vi "fpga_Reporting Rate Error Check (M Class).vi"(10 "reporting rate":i16, 11 "nominal frequency":enum16{"50 Hz", "60 Hz"}(ring)) -> (3 "error":i32)   [LabVIEW 2013, in "NI_EP_PMU_FPGA.lvlib"]
uses:
  <vilib>/addons/Electrical Power/PMU/NI_EP_PMU_FPGA.lvlib
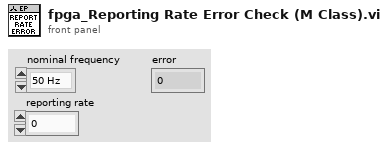
[diagram p1: front panel]
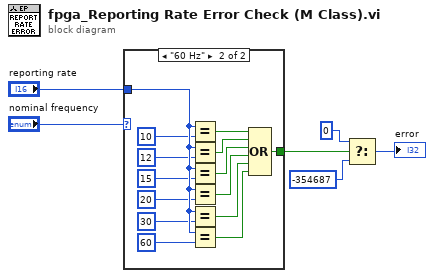
[diagram p0: block diagram]
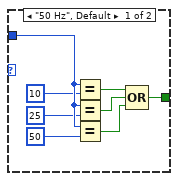
[diagram p2: hidden frame]
diagram:
  n1 = case shown="\"60 Hz\"" "nominal frequency" {
    tunnel: "reporting rate" -> [w11 w24]
    tunnel: [w10 w25] -> w4
    frame "50 Hz", Default {
      n2 = Equal?(x=w11, y=i16 10 ("reporting rate")) -> (x = y?=w14:bool)
      n3 = Equal?(x=w11, y=i16 25 ("reporting rate")) -> (x = y?=w13:bool)
      n4 = Equal?(x=w11, y=i16 50 ("reporting rate")) -> (x = y?=w12:bool)
      n5 = Compound Arithmetic op=OR(w14, w13, w12) -> (w10:bool)
    }
    frame "60 Hz" {
      n6 = Equal?(x=w24, y=i16 10 ("reporting rate")) -> (x = y?=w28:bool)
      n7 = Equal?(x=w24, y=i16 12 ("reporting rate")) -> (x = y?=w27:bool)
      n8 = Equal?(x=w24, y=i16 15 ("reporting rate")) -> (x = y?=w26:bool)
      n9 = Equal?(x=w24, y=i16 20 ("reporting rate")) -> (x = y?=w23:bool)
      n10 = Equal?(x=w24, y=i16 30 ("reporting rate")) -> (x = y?=w22:bool)
      n11 = Equal?(x=w24, y=i16 60 ("reporting rate")) -> (x = y?=w21:bool)
      n12 = Compound Arithmetic op=OR(w28, w27, w26, w23, w22, w21) -> (w25:bool)
    }
  }
  n13 = Select(t=0 ("error code (0)"), s=w4, f=-354687 ("error code (0)")) -> (s? t:f=→"error":i32)
